vi "Destroy.vi"(8 "error in":errorcluster, 11 "Logger in":refnum<class "Logger.lvclass">) -> (0 "error out":errorcluster, 3 "Logger out":refnum<class "Logger.lvclass">)   [LabVIEW 2016, in "hse-logger.lvlib" / "Logger.lvclass"]
doc: "Closes all handlers and removes them from the logger."
uses:
  Logger.lvclass
  Handler/Handler.lvclass
  Logger.lvclass/Logger.ctl
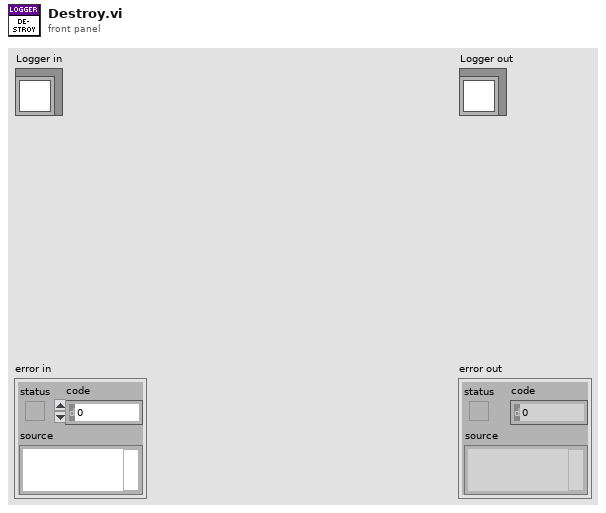
[diagram p1: front panel]
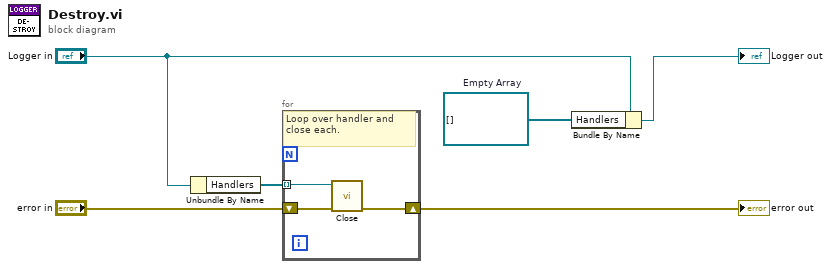
[diagram p0: block diagram]
diagram:
  w1 = refnum<class "Handler.lvclass">[] []  # Empty Array
  n1 = Unbundle By Name("Logger in") -> ("Handlers"=w3:refnum<class "Handler.lvclass">[])
  n2 = for {
    tunnel: w3 -> [w9] mode=indexing
    shift-right: [w7] -> w2
    shift-left: "error in" -> [w8]
    # "Loop over handler and close each."
    n3 = call-dynamic "Close.vi"("error in"=w8, "Handler in"=w9) -> ("error out"=w7:errorcluster)  [unwired: 8 in, 1 out]
  }
  "error out" <- w2
  n4 = Bundle By Name(cluster="Logger in", "Handlers"=w1) -> (→"Logger out":refnum<class "Logger.lvclass">)
